vi "ITR LP order 2.vi"(7 "input":dbl format="%.2f", 13 "corner period (steps)":dbl(slide)=10.237739663395852 scale=1.0..1000.0) -> (8 "output":dbl format="%.2f")   [LabVIEW 2016]
doc: "Modular ITR second order low pass filter with internal shift registers.\n\nAlexis Lopez\nP350\nCSUSB Physics"
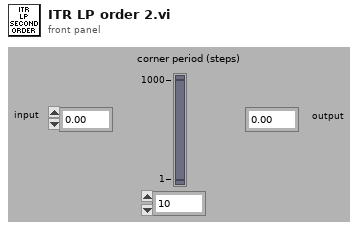
[diagram p1: front panel]
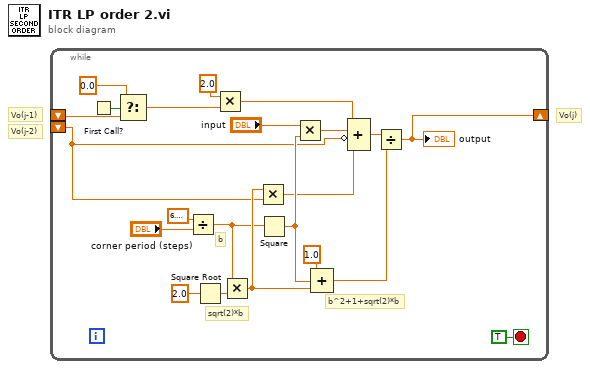
[diagram p0: block diagram]
diagram:
  # "Vo(j-2)"
  # "Vo(j-1)"
  # "Vo(j)"
  n1 = while {
    shift-left: _ -> [w13]
    shift-right: [w15] -> _
    shift-left: _ -> [w2]
    stop <- TRUE stop-if-true
    # "sqrt(2)*b"
    # "b^2+1+sqrt(2)*b"
    # "b"
    n2 = First Call?() -> (First Call?: T/F=w11:bool)
    n3 = Select(t=0.0, s=w11, f=w13) -> (s? t:f=w9:dbl)
    n4 = Divide(x=6.283185307179586, y="corner period (steps)") -> (x/y=w3:dbl)
    n5 = Square Root(x=2.0) -> (sqrt(x)=w4:dbl)
    n6 = Multiply(x=2.0, y=w9) -> (x*y=w10:dbl)
    n7 = Multiply(x=w3, y=w4) -> (x*y=w5:dbl)
    n8 = Multiply(x=w5, y=w2) -> (x*y=w1:dbl)
    n9 = Square(x=w3) -> (x^2=w6:dbl)
    n10 = Multiply(x="input", y=w6) -> (x*y=w14:dbl)
    n11 = Compound Arithmetic op=ADD(1.0, w6, w5) -> (w16:dbl)
    n12 = Compound Arithmetic op=ADD(w10, w14, invert w2, w1) -> (w17:dbl)
    n13 = Divide(x=w17, y=w16) -> (x/y=w15:dbl)
    "output" <- w15
  }
